vi "IR AOM freq to word.vi"(1 "Frequency In (MHz)":dbl) -> (0 "Frequency Word Out (double)":dbl format="%#_16e")   [LabVIEW 2014]
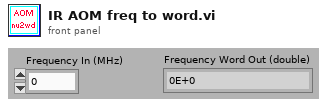
[diagram p1: front panel]
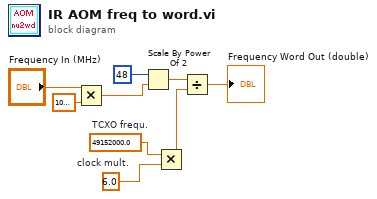
[diagram p0: block diagram]
diagram:
  w7 = 6.0  # clock mult.
  w8 = 49152000.0  # TCXO frequ.
  n1 = Multiply(x="Frequency In (MHz)", y=1000000.0) -> (x*y=w4:dbl)
  n2 = Scale By Power Of 2(n=48, x=w4) -> (x*2^n=w9:dbl)
  n3 = Multiply(x=w8, y=w7) -> (x*y=w6:dbl)
  n4 = Divide(x=w9, y=w6) -> (x/y=→"Frequency Word Out (double)":dbl)
